vi "Read Adu232.vi"(6 "#BytesToRead":u32, 7 "Timeout":u32, 8 "error in (no error)":errorcluster, 11 "RS232 handle":u32) -> (0 "error out":errorcluster, 1 "Read Buffer":string, 2 "function return":i32, 3 "RS232 handle out":u32, 4 "#BytesRead":u32)   [LabVIEW 2015, in "AduHid.lvlib"]
doc: "int __stdcall ReadAdu232(void * hRS232,\n void * lpBuffer,\n unsigned long nNumberOfBytesToRead,\n unsigned long * lpNumberOfBytesRead,\n unsigned long iTimeout);"
uses:
  AduHid.lvlib
  AduHid.dll
  Windows/SysWOW64/kernel32.dll
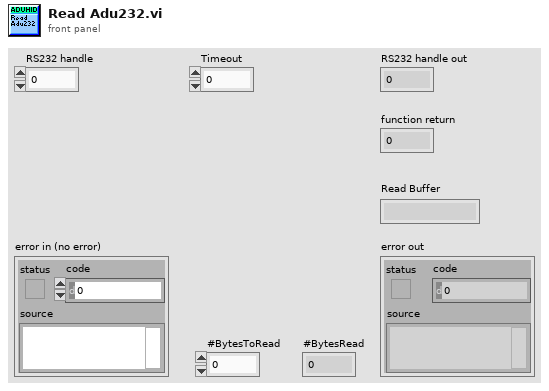
[diagram p1: front panel]
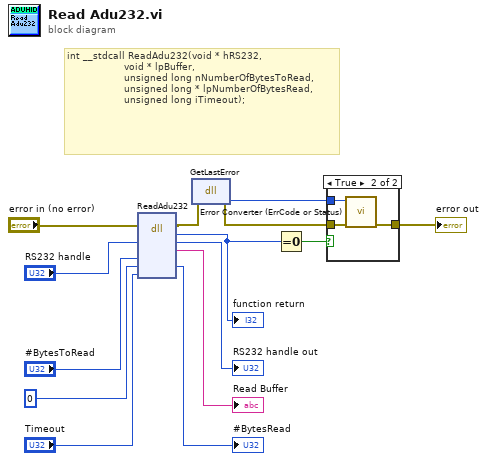
[diagram p0: block diagram]
diagram:
  # "int __stdcall ReadAdu232(void * hRS232,\n                   void * lpBuffer,\n                   unsigned long nNumberOfBytesToRead,\n                   unsigned long * lpNumberOfBytesRead,\n                   unsigned long iTimeout);"
  n1 = dll-call lib="C:/Projects/CBTF Modules/Libraries/Ontrak ADU/API/AduHid.*" fn="ReadAdu232"(error in="error in (no error)", "RS232 handle"="RS232 handle", "#BytesToRead"="#BytesToRead", "#BytesRead"=u32 0, "Timeout"="Timeout") -> (error out=w3:errorcluster, "return type"=w1:i32, "RS232 handle"=→"RS232 handle out":u32, "Read Buffer"=→"Read Buffer":string, "#BytesRead"=→"#BytesRead":u32)  [unwired: 5 in, 1 out]
  "function return" <- w1
  n2 = dll-call lib="C:/Windows/SysWOW64/kernel32.dll" fn="GetLastError"(error in=w3) -> (error out=w6:errorcluster, "return type"=w5:u32)  [unwired: 2 in, 1 out]
  n3 = Equal To 0?(x=w1) -> (x = 0?=w4:bool)
  n4 = case shown="True" w4 {
    tunnel: [w15 w18] -> w2
    tunnel: w6 -> [w15 w17]
    tunnel: w5 -> [_ w16]
    frame False {
    }
    frame True {
      n5 = call "Error Converter (ErrCode or Status).vi"("error in (no error)"=w17, "last error"=w16) -> ("error out"=w18:errorcluster)  [unwired: 9 in]
    }
  }
  "error out" <- w2
